vi "Write Reentrant_.vi"(8 "error in (no error)":errorcluster, 10 "Reentrant?":bool, 11 "VI in":refnum<class "VI.lvclass">) -> (0 "error out":errorcluster, 3 "VI out":refnum<class "VI.lvclass">)   [LabVIEW 2020, in "VI Properties Editor.lvlib" / "VI.lvclass"]
doc: "Gets or sets whether reentrancy is enabled for the VI."
uses:
  VI.lvclass
  VI.lvclass/VI.ctl
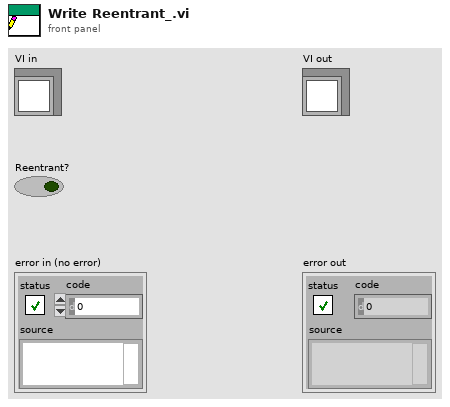
[diagram p1: front panel]
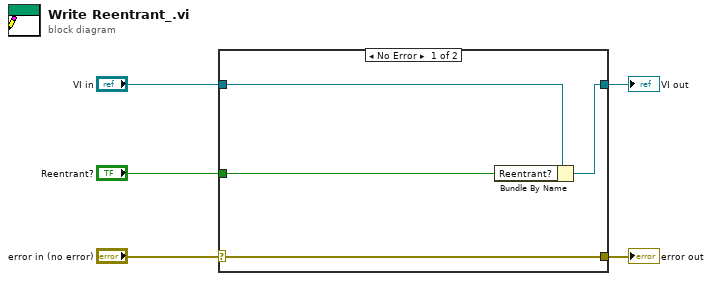
[diagram p0: block diagram]
diagram:
  n1 = case shown="No Error" "error in (no error)" {
    selector: "error in (no error)" -> [w9 w10]
    tunnel: [w9 w10] -> w4
    tunnel: [w7 w11] -> w2
    tunnel: "VI in" -> [w8 w11]
    tunnel: "Reentrant?" -> [w6 _]
    frame No Error {
      n2 = Bundle By Name(cluster=w8, "Reentrant?"=w6) -> (w7:refnum<class "VI.lvclass">)
    }
    frame Error {
    }
  }
  "error out" <- w4
  "VI out" <- w2
